vi "CRC.vi"(2 "Size":u8, 3 "Offset":i16, 4 "Data":refnum<k21>) -> (0 "CRC Lo":u8, 1 "CRC Hi":u8)   [LabVIEW 2018, in "Modbus_Processing_Unit.lvlib"]
uses:
  Modbus_Processing_Unit.lvlib
  <vilib>/rvi/Emulation/niFpgaSctlEmulationGetInTimedLoop.vi
  <vilib>/Utility/error.llb/Clear Errors.vi
  <vilib>/rvi/DataTransferAndStorage/Container/Common/niFpgaContainerExecOnDevCompGetState.vi
  <vilib>/rvi/Emulation/niFpgaEmulationIsFPGAContextNoSignature.vi
  <vilib>/rvi/DataTransferAndStorage/Container/Common/niFpgaContainerGetUniqueNameForEmu.vi
  <vilib>/rvi/Emulation/niFpgaProcessEmulError.vi
  <vilib>/rvi/errors/nirviReportUnexpectedCaseInternalError (U32).vi
  <vilib>/rvi/Memory/Memory_Emulation/niFpgaMemoryEmulationCacheClearOnFirstRun.vi
  <vilib>/rvi/Memory/Memory_Emulation/nirvimemoryEmulationManagerCache_MakeExclusive.vi
  <vilib>/rvi/Memory/Memory_Emulation/niFpgaMemoryEmulationValidateCache.vi
  <vilib>/rvi/Memory/Memory_Emulation/nirvimemoryEmulationManagerCache_InsertValue.vi
  <vilib>/rvi/Memory/Memory_Emulation/nirvimemoryEmulationManagerCache_ReleaseExclusive.vi
  <vilib>/rvi/Memory/Memory_Emulation/nirvimemoryEmulationManagerCache_GetValue.vi
  <vilib>/rvi/Memory/Memory_Emulation/nirvimemoryEmulationManagerCache_SetValue.vi
  <vilib>/rvi/Emulation/niFpgaSctlEmulationResourceMgr.vi
  <vilib>/rvi/DataTransferAndStorage/Container/XNode/niFpgaContainer.xnode
  <vilib>/rvi/Memory/Memory_Emulation/niFpgaMemoryEmulationRefIn.vi
panel:
  # "Calculates ModBus 16 bit CRC\n\nInput is array of uint8 values. Output is two\nuint8 values, representing CRC."
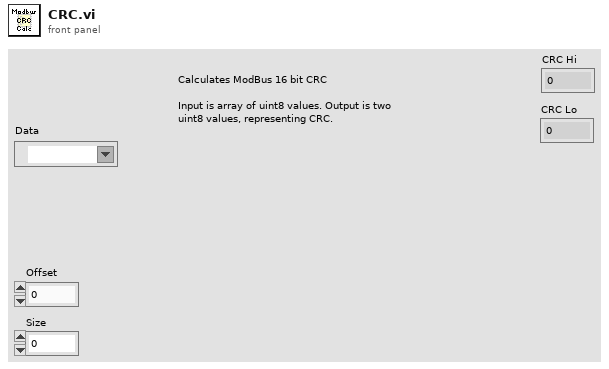
[diagram p1: front panel]
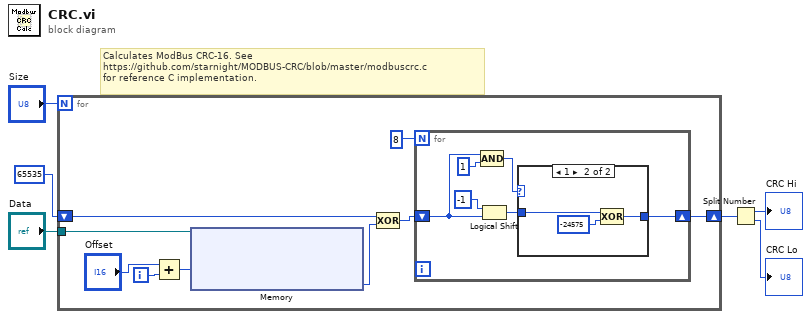
[diagram p0: block diagram]
diagram:
  # "Calculates ModBus CRC-16. See \nhttps://github.com/starnight/MODBUS-CRC/blob/master/modbuscrc.c\nfor reference C implementation."
  n1 = for {
    N: "Size" -> [_]
    tunnel: "Data" -> [w9]
    shift-right: [w10] -> w1
    shift-left: u16 65535 -> [w15]
    i -> [w12]
    n2 = Add(x="Offset", y=w12) -> (x+y=w8:i32)
    n3 = xnode "Memory"("Address"=w8, "Memory In"=w9) -> ("Data"=w7:u8)  [unwired: 1 out]
    n4 = Compound Arithmetic op=XOR(w15, w7) -> (w13:u16)
    n5 = for {
      N: i16 8 -> [_]
      shift-right: [w18] -> w10
      shift-left: w13 -> [w19]
      n6 = Logical Shift(y=i16 -1, x=w19) -> (x << y=w16:u16)
      n7 = Compound Arithmetic op=AND(w19, i16 1) -> (w21:u16)
      n8 = case shown="1" w21 {
        tunnel: [w22 w25] -> w18
        tunnel: w16 -> [w22 w23]
        frame 0, Default {
        }
        frame 1 {
          n9 = Compound Arithmetic op=XOR(w23, i16 -24575) -> (w25:u16)
        }
      }
    }
  }
  n10 = Split Number(x=w1) -> (hi(x)=→"CRC Hi":u8, lo(x)=→"CRC Lo":u8)
